vi "configure.vi"(8 "error in (no error)":errorcluster, 11 "GenericPlugin in":refnum<class "FPGAWrapperMH120124RAPS_PXI7813R.lvclass">) -> (0 "error out":errorcluster, 3 "GenericPlugin out":refnum<class "FPGAWrapperMH120124RAPS_PXI7813R.lvclass">)   [LabVIEW 2010, in "FPGAWrapperMH120124RAPS_PXI7813R.lvclass"]
doc: "The dynamic dispatch version of this VI loads and displays the configuration file associated with the plug-in object. The user modify and save the configuration data."
uses:
  FPGAWrapperMH120124RAPS_PXI7813R.lvclass
  fpgaVIsAndControls/DDS_board_init_cluster.ctl
  fpgaVIsAndControls/inverse_enum.ctl
  FPGAWrapperMH120124RAPS_PXI7813R.lvclass/FPGAWrapperMH120124RAPS_PXI7813R.ctl
  common/classes/GenericComponent/GenericComponent/GenericComponent.lvclass
panel:
  in  "cancel":bool
  in  "save":bool
  out "Configuration name":string
  in  "Tab Control":T1(tab)
  in  "AOD center frequency":dbl[unit]=94000000.0
  in  "AOD Bandwidth":dbl[unit]=34000000.0
  in  "inverse?":T2
  in  "OSK select":bool=TRUE
  in  "AOD equilibration time":dbl[unit]=7e-06
  in  "AOD lag iterations":i32
  in  "DDS board initialization parameters":T3={"Bypass PLL"=FALSE, "PLL Range"=TRUE, "Update Clock"=FALSE, "Triangle "=FALSE, "SDO Active"=FALSE, "LSB First"=FALSE, "OSK Int"=FALSE, "Output Shaped Keying Enable"=TRUE, "Bypass Sinc"=FALSE, "Digital Part"=TRUE, "OutPut DAC"=TRUE, "Control DAC"=TRUE, "Comparator"=FALSE, "Modus"=0, "Multiplier Value"=15} {"Modus" scale=0.0..4.0}
  # "Configure FPGAWrapperRAPS"
  # "The TrajectoryMH100122AODRAPS component controls the random access pattern scanning trajectory for the FPGA. \n\nEach FPGA controls the home built direct digital synthesizer (DDS) board that synthesizes the wave forms for the acousto-optic deflectors (AOD)."
  # "Settings for the direct digital synthesizer and acousto-optic de-flectors. See wiki page and manuals for standard values."
  # "FSK"
  # "Ramped"
  # "FSK"
  # "Chirp Modus"
  # "Unramped"
  # "BPSK"
  # "Single Tone"
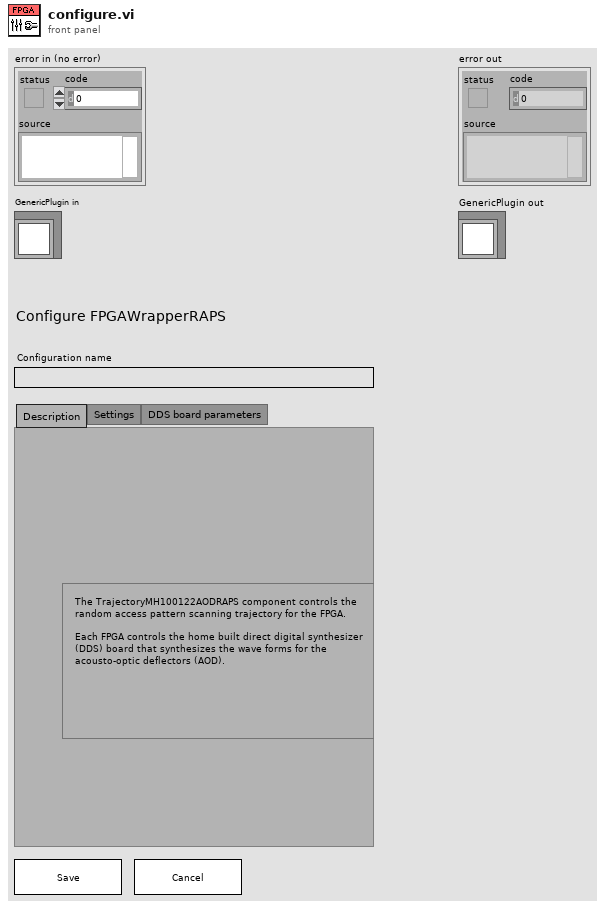
[diagram p1: front panel]
types:
  T1 = enum32{"Description", "Settings", "DDS board parameters"}
  T2 = typedef "inverse_enum.ctl" = enum16{"normal", "x inversed", "y inversed", "x & y inversed"}
  T3 = typedef "DDS_board_init_cluster.ctl" = cluster{"Bypass PLL":bool, "PLL Range":bool, "Update Clock":bool, "Triangle ":bool, "SDO Active":bool, "LSB First":bool, "OSK Int":bool, "Output Shaped Keying Enable":bool, "Bypass Sinc":bool, "Digital Part":bool, "OutPut DAC":bool, "Control DAC":bool, "Comparator":bool, "Modus":u8, "Multiplier Value":u8}
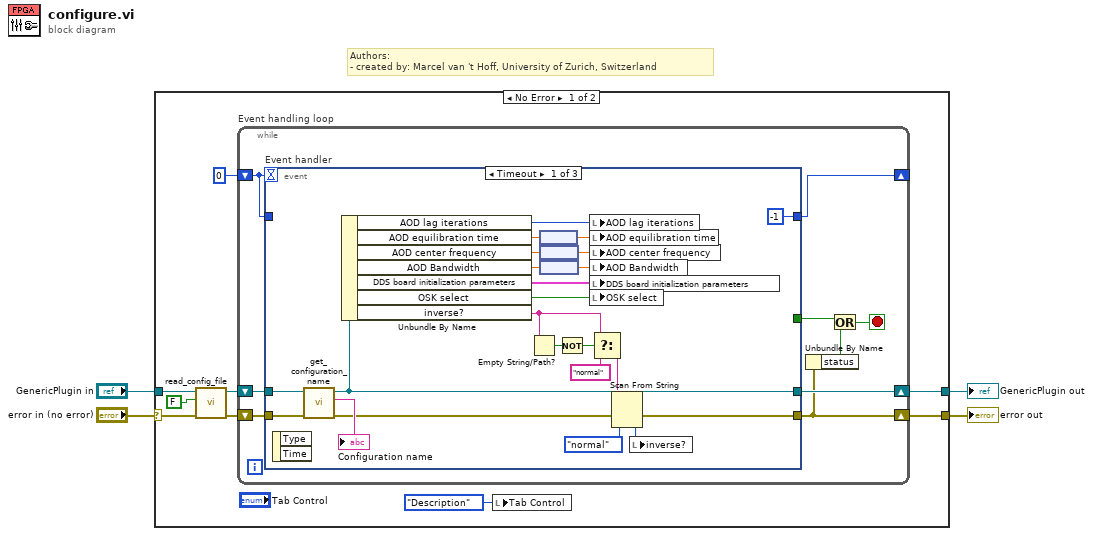
[diagram p0: block diagram]
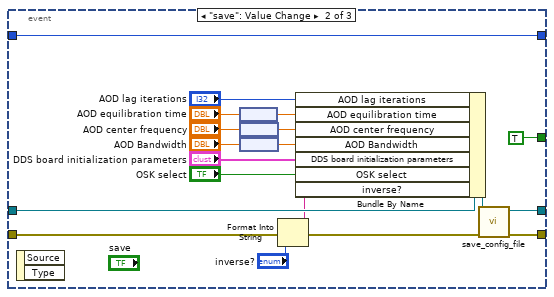
[diagram p2: hidden frame]
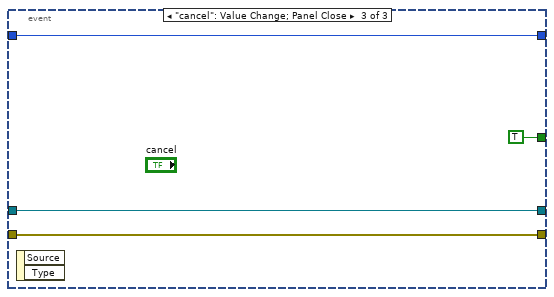
[diagram p3: hidden frame]
diagram:
  # "Authors: \n- created by: Marcel van 't Hoff, University of Zurich, Switzerland"
  n1 = case shown="No Error" "error in (no error)" {
    selector: "error in (no error)" -> [w10 w70]
    tunnel: [w12 w70] -> w2
    tunnel: [w11 w69] -> w1
    tunnel: "GenericPlugin in" -> [w8 w69]
    frame No Error {
      n2 = call-dynamic "read_config_file.vi"("error in (no error)"=w10, "force load?"=FALSE, "GenericPlugin in"=w8) -> ("error out"=w9:errorcluster, "GenericPlugin out"=w7:refnum<class "FPGAWrapperMH120124RAPS_PXI7813R.lvclass">)  [unwired: 7 out]
      n3 = while "Event handling loop" {
        shift-right: [w20] -> _
        shift-left: 0 -> [w21]
        shift-right: [w17] -> w12
        shift-left: w9 -> [w22]
        shift-right: [w18] -> w11
        shift-left: w7 -> [w19]
        stop <- w15 stop-if-true
        n4 = event "Event handler" shown="[0] Timeout" {
          selector: _ -> [_ _ _]
          dyn-events: _ -> [_ _ _]
          timeout: w21 -> [_ _ _]
          tunnel: w22 -> [w44 w55 w67]
          tunnel: [-1 w64 w68] -> w20
          tunnel: w21 -> [_ w64 w68]
          tunnel: [w35 w63 w67] -> w17
          tunnel: [_ TRUE TRUE] -> w14
          tunnel: w19 -> [w43 w58 w65]
          tunnel: [w39 w62 w65] -> w18
          event Timeout {
            n5 = event-data() -> ()  [unwired: 3 out]
            n6 = call "get_configuration_name.vi"("error in (no error)"=w44, "GenericPlugin.lvclass in"=w43) -> ("error out"=w36:errorcluster, "configuration name"=→"Configuration name":string, "GenericPlugin.lvclass out"=w39:refnum<class "FPGAWrapperMH120124RAPS_PXI7813R.lvclass">)  [unwired: 7 in]
            n7 = Unbundle By Name(w39) -> ("AOD lag iterations"=w33:i32, "AOD equilibration time"=w38:dbl, "AOD center frequency"=w26:dbl, "AOD Bandwidth"=w25:dbl, "DDS board initialization parameters"=w40:T3, "OSK select"=w41:bool, "inverse?"=w29:string)
            n8 = Empty String/Path?(string/path=w29) -> (empty?=w32:bool)
            n9 = node(w38) -> (w27:dbl[unit])
            n10 = node(w26) -> (w23:dbl[unit])
            n11 = node(w25) -> (w24:dbl[unit])
            n12 = Not(x=w32) -> (.not. x?=w31:bool)
            n13 = local write "AOD lag iterations"(w33) -> ()
            n14 = local write "AOD equilibration time"(w27) -> ()
            n15 = local write "AOD center frequency"(w23) -> ()
            n16 = local write "AOD Bandwidth"(w24) -> ()
            n17 = local write "DDS board initialization parameters"(w40) -> ()
            n18 = local write "OSK select"(w41) -> ()
            n19 = Select(t=w29, s=w31, f="normal") -> (s? t:f=w28:string)
            n20 = Scan From String(input string=w28, error in=w36, default 1=inverse_enum."normal" ("inverse?")) -> (error out=w35:errorcluster, output 1=w37:T2)  [unwired: 2 in, 2 out]
            n21 = local write "inverse?"(w37) -> ()
          }
          event "save": Value Change {
            n22 = event-data() -> ()  [unwired: 3 out]
            n23 = node("AOD equilibration time") -> (w50:dbl)
            n24 = node("AOD center frequency") -> (w47:dbl)
            n25 = node("AOD Bandwidth") -> (w46:dbl)
            n26 = Format Into String(error in=w55, "inverse?") -> (resulting string=w56:string, error out=w54:errorcluster)  [unwired: 2 in]
            n27 = Bundle By Name(cluster=w58, "AOD lag iterations"="AOD lag iterations", "AOD equilibration time"=w50, "AOD center frequency"=w47, "AOD Bandwidth"=w46, "DDS board initialization parameters"="DDS board initialization parameters", "OSK select"="OSK select", "inverse?"=w56) -> (w57:refnum<class "FPGAWrapperMH120124RAPS_PXI7813R.lvclass">)
            n28 = call-dynamic "save_config_file.vi"("error in (no error)"=w54, "GenericPlugin in"=w57) -> ("error out"=w63:errorcluster, "GenericPlugin out"=w62:refnum<class "FPGAWrapperMH120124RAPS_PXI7813R.lvclass">)  [unwired: 2 in, 6 out]
          }
          event "cancel": Value Change; Panel Close {
            n29 = event-data() -> ()  [unwired: 3 out]
          }
        }
        n30 = Unbundle By Name(w17) -> ("status"=w16:bool)
        n31 = Or(x=w14, y=w16) -> (x .or. y?=w15:bool)
      }
      n32 = local write "Tab Control"(T1."Description" ("Tab Control")) -> ()
    }
    frame Error {
    }
  }
  "error out" <- w2
  "GenericPlugin out" <- w1
